vi "重构模块.vi"(0 "重建方法":u16(ring) items=["二阶重构", "压缩感知"], 1 "采样次数":i32, 2 "图像1024一维数组":dbl[](array[numeric]), 3 "簇":T1, 4 "少量采样数据量M":i32 min=0 max=100000 step=1) -> (5 "重构图像":dbl[][](array[numeric]))   [LabVIEW 2018]
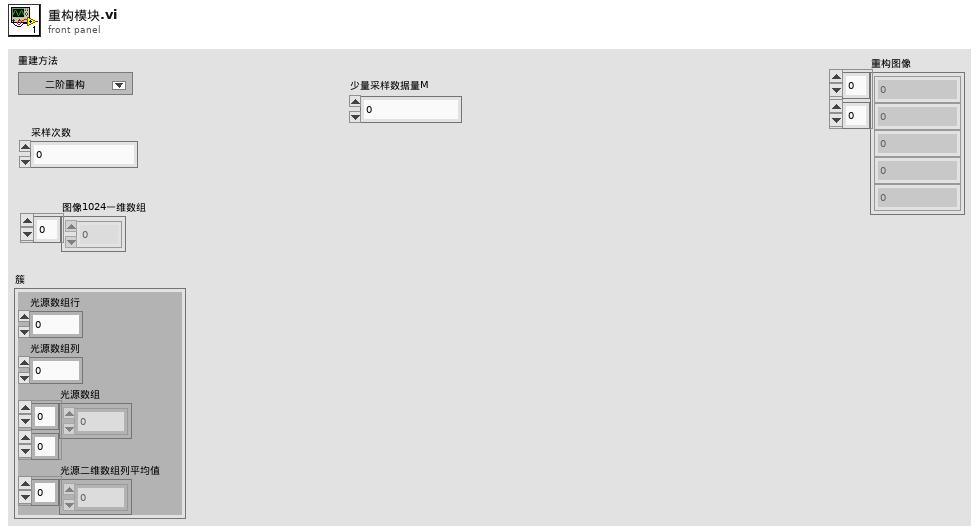
[diagram p1: front panel]
types:
  T1 = cluster{"光源数组行":i32, "光源数组列":i32, "光源数组":dbl[][], "光源二维数组列平均值":dbl[]}
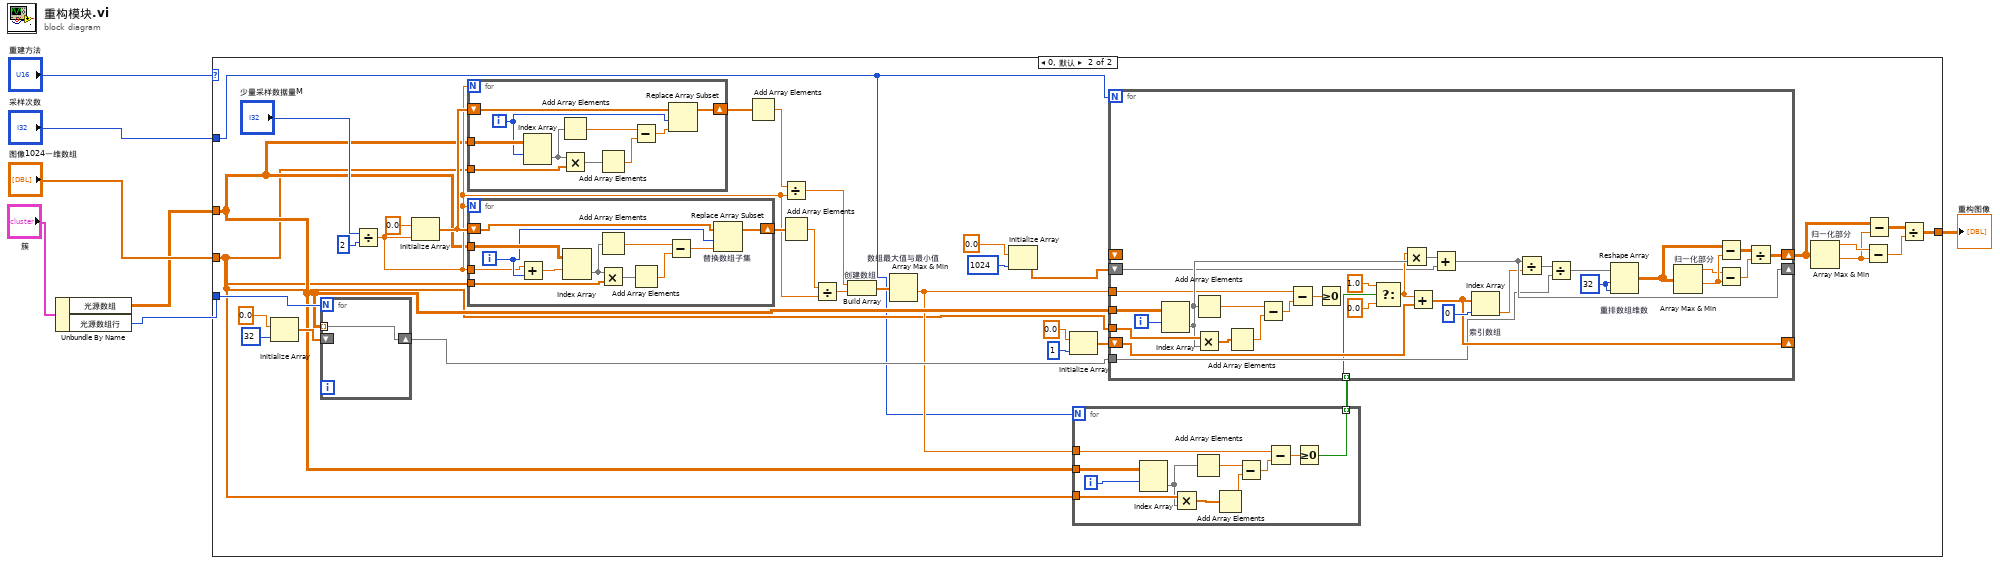
[diagram p0: block diagram]
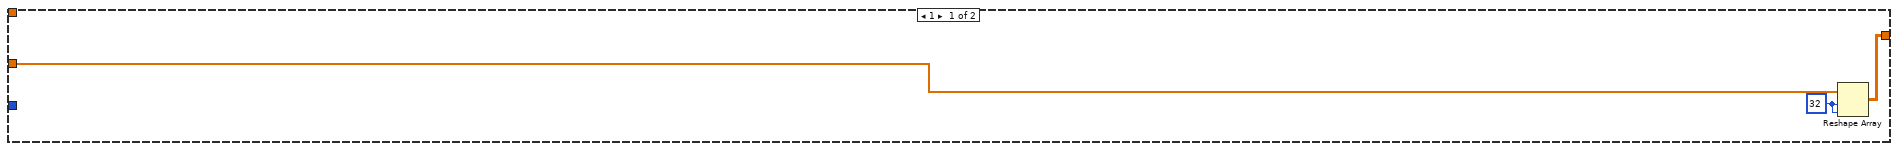
[diagram p2: hidden frame]
diagram:
  n1 = Unbundle By Name("簇") -> ("光源数组"=w2:dbl[][], "光源数组行"=w1:i32)
  n2 = case shown="0, 默认" "重建方法" {
    tunnel: "采样次数" -> [_ w12]
    tunnel: w2 -> [_ w15]
    tunnel: "图像1024一维数组" -> [w9 w13]
    tunnel: [w8 w34] -> w6
    tunnel: w1 -> [_ w20]
    frame 1 {
      w10 = 32
      n3 = Reshape Array(w9, w10, w10) -> (w8:dbl[][])
    }
    frame 0, Default {
      n4 = Initialize Array(0.0, 32) -> (w17:dbl[])
      n5 = for {
        N: w20 -> [_]
        shift-right: [w56] -> w16
        shift-left: w17 -> [_]
        tunnel: w15 -> [w56] mode=indexing
      }
      n6 = Divide(x="少量采样数据量M", y=2) -> (x/y=w21:dbl)
      n7 = Initialize Array(0.0 ("元素"), w21) -> (w23:dbl[])
      n8 = for "For循环" {
        N: w21 -> [_]
        tunnel: w15 -> [w78]
        tunnel: w13 -> [w69]
        shift-right: [w70] -> w30
        shift-left: w23 -> [w73]
        i -> [w71]
        n9 = Index Array(array=w78, index (row)=w71) -> (element=w76:dbl[])  [unwired: 1 in]
        n10 = Add Array Elements(numeric array=w76) -> (sum=w74:dbl)
        n11 = Multiply(x=w76, y=w69) -> (x*y=w77:dbl[])
        n12 = Add Array Elements(numeric array=w77) -> (sum=w75:dbl)
        n13 = Subtract(x=w74, y=w75) -> (x-y=w72:dbl)
        n14 = Replace Array Subset(array=w73, new element=w72, index=w71) -> (w70:dbl[])
      }
      n15 = for {
        N: w21 -> [_]
        tunnel: w15 -> [w68]
        shift-right: [w61] -> w28
        shift-left: w23 -> [w63]
        tunnel: w13 -> [w58]
        tunnel: w21 -> [w57]
        i -> [w59]
        n16 = Add(x=w57, y=w59) -> (x+y=w60:dbl)
        n17 = Index Array(array=w68, index (row)=w60) -> (element=w66:dbl[])  [unwired: 1 in]
        n18 = Add Array Elements(numeric array=w66) -> (sum=w64:dbl)
        n19 = Multiply(x=w66, y=w58) -> (x*y=w67:dbl[])
        n20 = Add Array Elements(numeric array=w67) -> (sum=w65:dbl)
        n21 = Subtract(x=w64, y=w65) -> (x-y=w62:dbl)
        n22 = Replace Array Subset "替换数组子集"(array=w63, new element=w62, index=w59) -> (w61:dbl[])
      }
      n23 = Add Array Elements(numeric array=w30) -> (sum=w29:dbl)
      n24 = Divide(x=w29, y=w21) -> (x/y=w25:dbl)
      n25 = Add Array Elements(numeric array=w28) -> (sum=w27:dbl)
      n26 = Divide(x=w27, y=w21) -> (x/y=w24:dbl)
      n27 = Build Array "创建数组"(w25, w24) -> (w26:dbl[])
      n28 = Array Max & Min "数组最大值与最小值"(array=w26) -> (min value=w14:dbl)  [unwired: 3 out]
      n29 = Initialize Array(0.0 ("元素"), 1024 ("维数大小")) -> (w40:dbl[])
      n30 = Initialize Array(0.0 ("元素"), 1 ("维数大小")) -> (w39:dbl[])
      n31 = for {
        N: w12 -> [_]
        tunnel: w15 -> [w50]
        tunnel: w14 -> [w48]
        tunnel: w13 -> [w47]
        tunnel: [w45] -> w11 mode=indexing
        i -> [w49]
        n32 = Index Array(array=w50, index (row)=w49) -> (element=w46:dbl[])  [unwired: 1 in]
        n33 = Multiply(x=w47, y=w46) -> (x*y=w51:dbl[])
        n34 = Add Array Elements(numeric array=w46) -> (sum=w52:dbl)
        n35 = Add Array Elements(numeric array=w51) -> (sum=w53:dbl)
        n36 = Subtract(x=w52, y=w53) -> (x-y=w54:dbl)
        n37 = Subtract(x=w48, y=w54) -> (x-y=w55:dbl)
        n38 = Greater Or Equal To 0?(x=w55) -> (x >= 0?=w45:bool)
      }
      n39 = for {
        N: w12 -> [_]
        tunnel: w15 -> [w108]
        tunnel: w13 -> [w107]
        shift-right: [w95] -> _
        shift-left: w40 -> [w80]
        shift-right: [w91] -> _
        shift-left: w39 -> [w93]
        tunnel: w14 -> [w87]
        tunnel: w16 -> [w82]
        shift-right: [w81] -> w33
        shift-left: _ -> [_]
        tunnel: w11 -> [w79] mode=indexing
        i -> [w109]
        w101 = 32 ("维数大小")
        n40 = Index Array(array=w108, index (row)=w109) -> (element=w96:dbl[])  [unwired: 1 in]
        n41 = Add Array Elements(numeric array=w96) -> (sum=w90:dbl)
        n42 = Multiply(x=w107, y=w96) -> (x*y=w106:dbl[])
        n43 = Add Array Elements(numeric array=w106) -> (sum=w89:dbl)
        n44 = Subtract(x=w90, y=w89) -> (x-y=w88:dbl)
        n45 = Subtract(x=w87, y=w88) -> (x-y=w86:dbl)
        n46 = Greater Or Equal To 0?(x=w86) -> ()  [unwired: 1 out]
        n47 = Select(t=1.0, s=w79, f=0.0) -> (s? t:f=w83:dbl)
        n48 = Multiply(x=w83, y=w96) -> (x*y=w97:dbl[])
        n49 = Add(x=w83, y=w93) -> (x+y=w91:dbl[])
        n50 = Add(x=w97, y=w80) -> (x+y=w95:dbl[])
        n51 = Index Array "索引数组"(array=w91, index=0 ("索引")) -> (element=w92:dbl)
        n52 = Divide(x=w95, y=w92) -> (x/y=w98:dbl[])
        n53 = Divide(x=w98, y=w82) -> (x/y=w99:dbl[])
        n54 = Reshape Array "重排数组维数"(w99, w101, w101) -> (w100:dbl[][])
        n55 = Array Max & Min "归一化部分"(array=w100) -> (max value=w102:dbl, min value=w103:dbl)  [unwired: 2 out]
        n56 = Subtract(x=w100, y=w103) -> (x-y=w104:dbl[][])
        n57 = Subtract(x=w102, y=w103) -> (x-y=w105:dbl)
        n58 = Divide(x=w104, y=w105) -> (x/y=w81:dbl[][])
      }
      n59 = Array Max & Min "归一化部分"(array=w33) -> (max value=w38:dbl, min value=w37:dbl)  [unwired: 2 out]
      n60 = Subtract(x=w38, y=w37) -> (x-y=w35:dbl)
      n61 = Subtract(x=w33, y=w37) -> (x-y=w36:dbl[][])
      n62 = Divide(x=w36, y=w35) -> (x/y=w34:dbl[][])
    }
  }
  "重构图像" <- w6
